vi "Reset.vi"(8 "error in (no error)":errorcluster, 10 "Message in":refnum<class "ResetMessage.lvclass">, 11 "Autofocus in":refnum<class "Autofocus.lvclass">) -> (0 "error out":errorcluster, 3 "Autofocus out":refnum<class "Autofocus.lvclass">)   [LabVIEW 2012, in "Autofocus.lvclass"]
doc: "The reset method processes the command 'reset'. \n\nResets the internal state of the component (without performing a full initialisation). This could be resetting hardware, or private data to default values."
uses:
  Autofocus.lvclass
  <vilib>/Distrio/Murmex/ResetMessage/ResetMessage.lvclass
  <vilib>/Distrio/Murmex/Murmex/Murmex.lvclass
  Autofocus.lvclass/Autofocus.ctl
panel:
  # "This method is called when the RESET\ntrigger is sent. \n\nOverride this method when your component needs to\nrespond to this trigger. \n\nCall parent for proper implementation"
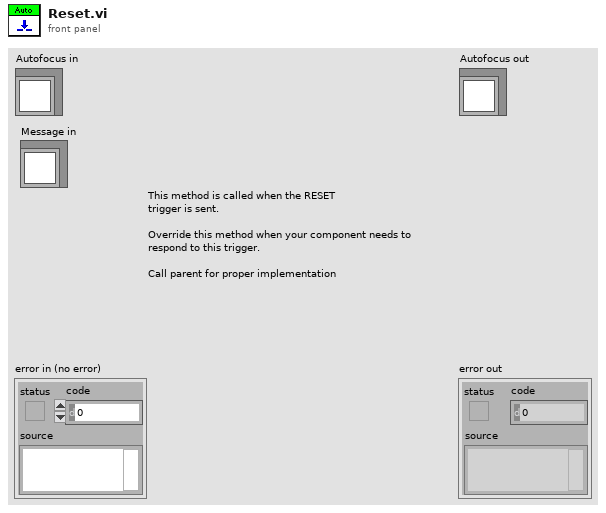
[diagram p1: front panel]
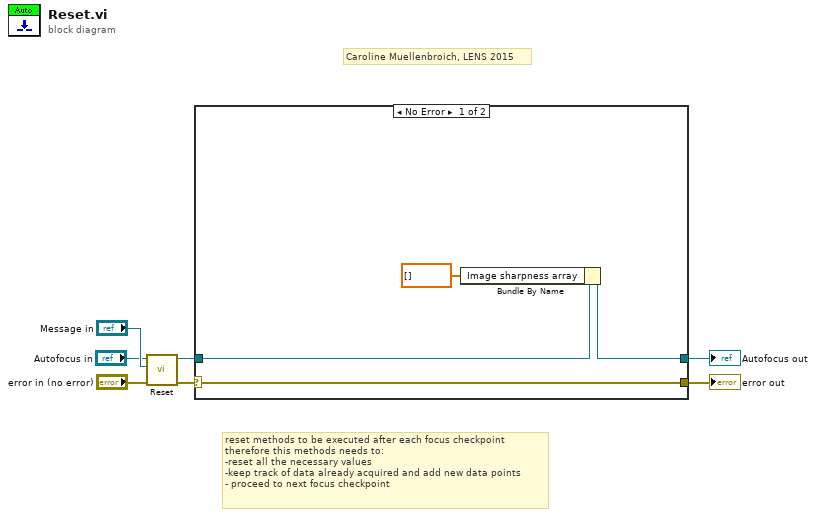
[diagram p0: block diagram]
diagram:
  # "reset methods to be executed after each focus checkpoint\ntherefore this methods needs to:\n-reset all the necessary values\n-keep track of data already acquired and add new data points\n- proceed to next focus checkpoint"
  # "Caroline Muellenbroich, LENS 2015"
  n1 = call-parent "Reset.vi"("error in (no error)"="error in (no error)", "Message in"="Message in", "Murmex in"="Autofocus in") -> ("error out"=w4:errorcluster, "Murmex out"=w2:refnum<class "Autofocus.lvclass">)  [unwired: 7 in]
  n2 = case shown="No Error" w4 {
    selector: w4 -> [w11 w13]
    tunnel: [w11 w13] -> w3
    tunnel: w2 -> [w10 w12]
    tunnel: [w9 w12] -> w1
    frame No Error {
      n3 = Bundle By Name(cluster=w10, "Image sharpness array"=dbl[] [] ("Runtime cluster.Checkpoint .Image sharpness array")) -> (w9:refnum<class "Autofocus.lvclass">)
    }
    frame Error {
    }
  }
  "error out" <- w3
  "Autofocus out" <- w1
